vi "Change Bit Value - Single.vi"(8 "error in (no error)":errorcluster, 9 "State":u8(ring) items=["0", "1", "Z", "L", "H", "X", "T", "V"], 10 "Bit":T4 items=["SDA", "SCL"], 11 "I2C waveform info":T1) -> (0 "error out":errorcluster, 3 "I2C waveform info out":T1)   [LabVIEW 2009, in "IDW.lvlib"]
doc: "Appends a single sample to the I2C waveform wherein one of the bus lines (SCL or SDA) changes value."
uses:
  IDW.lvlib
  _Typedefs/Channel Ring.ctl
  _Typedefs/Waveform info.ctl
  _Typedefs/Timing - ticks.ctl
  _Typedefs/Default transition action.ctl
  _Typedefs/Bit type.ctl
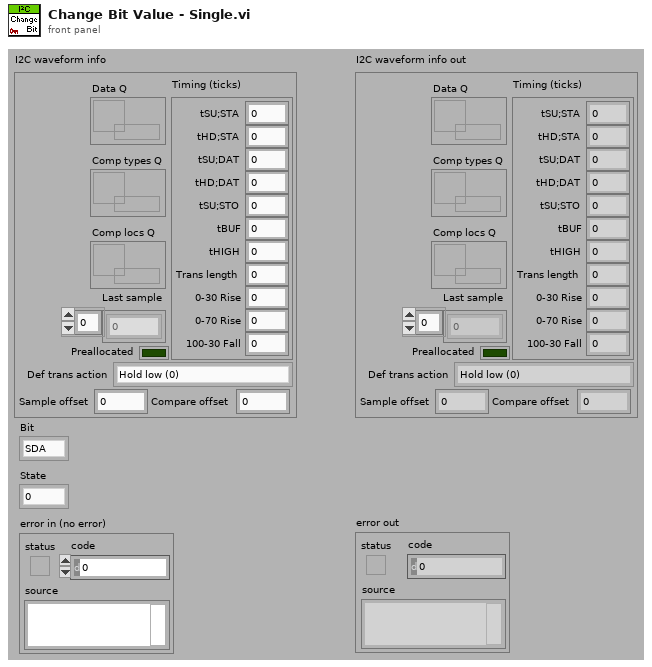
[diagram p1: front panel]
types:
  T1 = typedef "IDW.lvlib/Waveform info.ctl" = cluster{"Last sample":u8[], "Sample offset":u64, "Compare offset":u64, "Timing (ticks)":T2, "Preallocated":bool, "Def trans action":T3, "Data Q":refnum<queue>, "Comp types Q":refnum<queue>, "Comp locs Q":refnum<queue>}
  T2 = typedef "IDW.lvlib/Timing - ticks.ctl" = cluster{"tSU;STA":i32, "tHD;STA":i32, "tSU;DAT":i32, "tHD;DAT":i32, "tSU;STO":i32, "tBUF":i32, "tHIGH":i32, "Trans length":i32, "0-30 Rise":i32, "0-70 Rise":i32, "100-30 Fall":i32}
  T3 = typedef "IDW.lvlib/Default transition action.ctl" = enum16{"Hold low (0)", "Release (Z)", "Set up next value", "Hold previous value", "Preserve tHD;DAT and tSU;DAT"}
  T4 = typedef "IDW.lvlib/Channel Ring.ctl" = u16
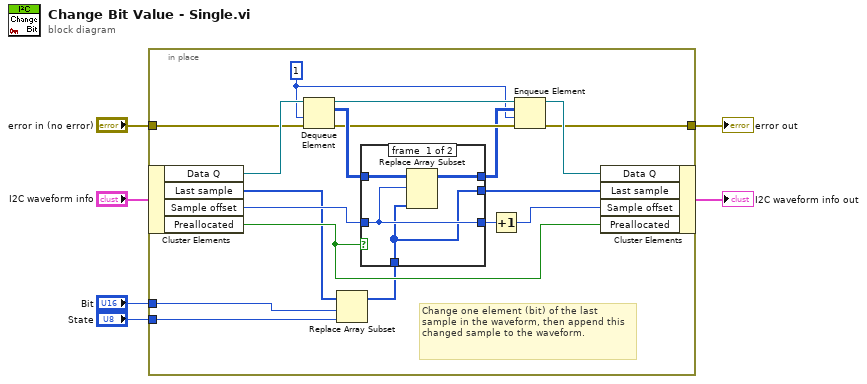
[diagram p0: block diagram]
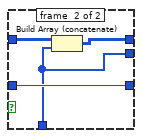
[diagram p2: hidden frame]
diagram:
  n1 = in-place {
    in-place-border: "Bit" -> [w17]
    in-place-border: "State" -> [w18]
    in-place-border: "error in (no error)" -> [w9]
    in-place-border: [w8] -> w1
    w7 = 1 ("timeout in ms (-1)")
    # "Change one element (bit) of the last sample in the waveform, then append this changed sample to the waveform."
    n2 = in-place-cluster #1("I2C waveform info") -> ("Data Q"=w24:refnum<queue>, "Last sample"=w15:u8[], "Sample offset"=w21:u64, "Preallocated"=w22:bool)
    n3 = Dequeue Element(queue=w24, timeout in ms (-1)=w7, error in (no error)=w9) -> (queue out=w13:refnum<queue>, element=w14:u8[][], error out=w12:errorcluster)  [unwired: 1 out]
    n4 = Replace Array Subset(array=w15, new element=w18, index=w17) -> (w16:u8[])
    n5 = case shown="False" w22 {
      tunnel: w14 -> [w28 w32]
      tunnel: [w25 w29] -> w23
      tunnel: [w27 w31] -> w11
      tunnel: w21 -> [w26 w30]
      tunnel: [w26 w30] -> w20
      tunnel: w16 -> [w25 w29]
      frame #0 {
        n6 = Replace Array Subset(array=w28, new element=w25, index (row)=w26) -> (w27:u8[][])  [unwired: 1 in]
      }
      frame #1 {
        n7 = Build Array (concatenate)(w32, w29) -> (w31:u8[][])
      }
    }
    n8 = Increment(x=w20) -> (x+1=w19:u64)
    n9 = Enqueue Element(queue=w13, element=w11, timeout in ms (-1)=w7, error in (no error)=w12) -> (queue out=w10:refnum<queue>, error out=w8:errorcluster)  [unwired: 1 out]
    n10 = in-place-cluster #1("Data Q"=w10, "Last sample"=w23, "Sample offset"=w19, "Preallocated"=w22) -> (→"I2C waveform info out":T1)
  }
  "error out" <- w1
